vi "New Item Status.vi"(8 "error in (no error)":errorcluster, 10 "Status":string, 11 "Bar in":refnum<class "Bar.lvclass">) -> (0 "error out":errorcluster, 3 "Bar out":refnum<class "Bar.lvclass">)   [LabVIEW 2015, in "Simple Progress Bar.lvlib" / "Bar.lvclass"]
doc: "Display a new <b>Status</b> text in the second progress bar indicator. Step progression is managed automatically with the items count declared with the New Job VI."
uses:
  Class/Bar.lvclass
  Class/Bar.lvclass/Bar.ctl
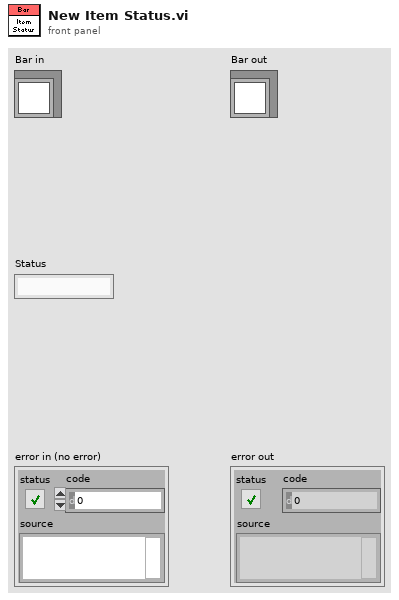
[diagram p1: front panel]
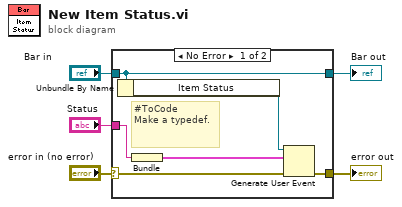
[diagram p0: block diagram]
diagram:
  n1 = case shown="No Error" "error in (no error)" {
    selector: "error in (no error)" -> [w10 w12]
    tunnel: "Bar in" -> [w8 w13]
    tunnel: [w8 w13] -> w3
    tunnel: [w9 w12] -> w2
    tunnel: "Status" -> [w7 _]
    frame No Error {
      # "#ToCode\nMake a typedef."
      n2 = Unbundle By Name(w8) -> ("Item Status"=w11:refnum<user-event>)
      n3 = Bundle("Status"=w7) -> (w6:cluster{"Status":string})  [unwired: 1 in]
      n4 = Generate User Event(user event=w11, event data cluster=w6, error in=w10) -> (error out=w9:errorcluster)  [unwired: 1 in, 1 out]
    }
    frame Error {
    }
  }
  "error out" <- w2
  "Bar out" <- w3
